vi "Initialize.vi"(7 "IP":string="//localhost", 8 "error in (no error)":errorcluster, 9 "Image Name":string="CH1", 10 "Night Directory:":string="C:\\Users\\observer\\Desktop\\Imagens", 11 "SPARC4_GUI in":refnum<class "SPARC4_GUI.lvclass">) -> (0 "error out":errorcluster, 3 "SPARC4_GUI out":refnum<class "SPARC4_GUI.lvclass">)   [LabVIEW 2018, in "SPARC4_GUI.lvclass"]
uses:
  SPARC4_GUI.lvclass
  Channel GUI/Channel GUI.lvclass
  Channel GUI/Channel GUI.lvclass/Channel GUI.ctl
  SPARC4_GUI.lvclass/SPARC4_GUI.ctl
  State Machine/State Machine.lvclass
panel:
  in  "Channel GUI.lvclass":refnum<class "Channel GUI.lvclass">
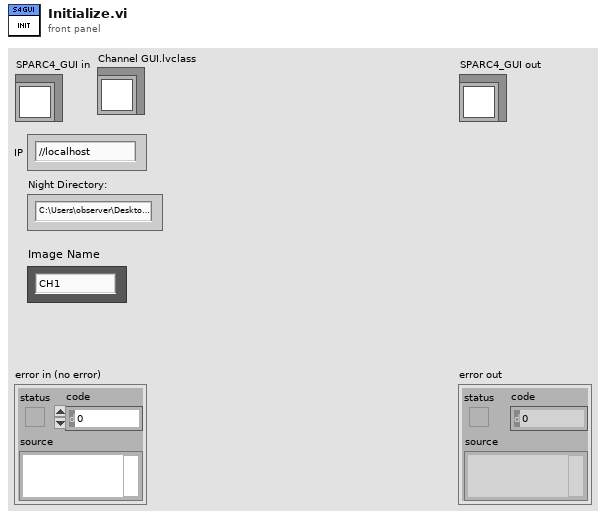
[diagram p1: front panel]
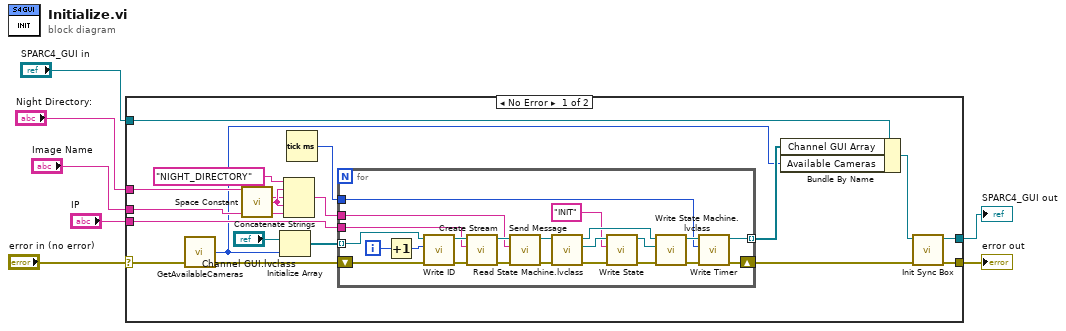
[diagram p0: block diagram]
diagram:
  n1 = case shown="No Error" "error in (no error)" {
    selector: "error in (no error)" -> [w18 w50]
    tunnel: [w10 w50] -> w6
    tunnel: [w11 w49] -> w4
    tunnel: "SPARC4_GUI in" -> [w15 w49]
    tunnel: "Image Name" -> [w23 _]
    tunnel: "Night Directory:" -> [w22 _]
    tunnel: "IP" -> [w17 _]
    frame No Error {
      n2 = call <userlib>:"GetAvailableCameras.vi"("error in (no error)"=w18) -> ("error out"=w19:errorcluster, "totalCameras"=w8:i32)  [unwired: 2 in, 1 out]
      n3 = call <vilib>:"Space Constant.vi"() -> ("String"=w24:string)
      n4 = Initialize Array("Channel GUI.lvclass", w8) -> (w20:refnum<class "Channel GUI.lvclass">[])
      n5 = Concatenate Strings("NIGHT_DIRECTORY" ("Message"), w24, w22, w24, w23) -> (w16:string)
      n6 = Tick Count (ms)() -> (millisecond timer value=w14:u32)
      n7 = for {
        shift-right: [w26] -> w9
        shift-left: w19 -> [w46]
        tunnel: w20 -> [w47] mode=indexing
        tunnel: w17 -> [w40]
        tunnel: w16 -> [w39]
        tunnel: w14 -> [w28]
        tunnel: [w27] -> w13 mode=indexing
        i -> [w48]
        n8 = Increment(x=w48) -> (x+1=w45:i32)
        n9 = call "Write ID.vi"("error in (no error)"=w46, "ID"=w45, "Channel GUI in"=w47) -> ("error out"=w44:errorcluster, "Channel GUI out"=w43:refnum<class "Channel GUI.lvclass">)  [unwired: 7 in]
        n10 = call "Create Stream.vi"("error in (no error)"=w44, "IP"=w40, "Channel GUI in"=w43) -> ("error out"=w41:errorcluster, "Channel GUI out"=w42:refnum<class "Channel GUI.lvclass">)  [unwired: 7 in]
        n11 = call "Send Message.vi"("error in (no error)"=w41, "Message"=w39, "Channel GUI in"=w42) -> ("error out"=w37:errorcluster, "Channel GUI out"=w38:refnum<class "Channel GUI.lvclass">)  [unwired: 7 in]
        n12 = call "Read State Machine.lvclass.vi"("error in (no error)"=w37, "Channel GUI in"=w38) -> ("error out"=w33:errorcluster, "State Machine.lvclass"=w36:refnum<class "State Machine.lvclass">, "Channel GUI out"=w34:refnum<class "Channel GUI.lvclass">)  [unwired: 7 in]
        n13 = call-dynamic "Write State.vi"("error in (no error)"=w33, "State"="INIT", "State Machine in"=w36) -> ("error out"=w32:errorcluster, "State Machine out"=w35:refnum<class "State Machine.lvclass">)  [unwired: 7 in]
        n14 = call "Write State Machine.lvclass.vi"("error in (no error)"=w32, "State Machine.lvclass"=w35, "Channel GUI in"=w34) -> ("error out"=w29:errorcluster, "Channel GUI out"=w30:refnum<class "Channel GUI.lvclass">)  [unwired: 7 in]
        n15 = call "Write Timer.vi"("error in (no error)"=w29, "Timer"=w28, "Channel GUI in"=w30) -> ("error out"=w26:errorcluster, "Channel GUI out"=w27:refnum<class "Channel GUI.lvclass">)  [unwired: 7 in]
      }
      n16 = Bundle By Name(cluster=w15, "Channel GUI Array"=w13, "Available Cameras"=w8) -> (w12:refnum<class "SPARC4_GUI.lvclass">)
      n17 = call "Init Sync Box.vi"("error in (no error)"=w9, "SPARC4_GUI in"=w12) -> ("error out"=w10:errorcluster, "SPARC4_GUI out"=w11:refnum<class "SPARC4_GUI.lvclass">)  [unwired: 8 in]
    }
    frame Error {
    }
  }
  "error out" <- w6
  "SPARC4_GUI out" <- w4
